vi "PLC WRITE DATA.vi"(8 "error in (no error)":errorcluster, 10 "cmd":string, 11 "TCP Network Connection in":refnum<k5>) -> (0 "error out":errorcluster, 3 "TCP Network Connection out":refnum<k5>)   [LabVIEW 2015]
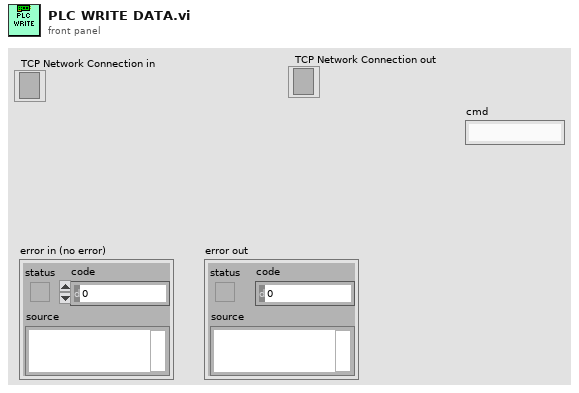
[diagram p1: front panel]
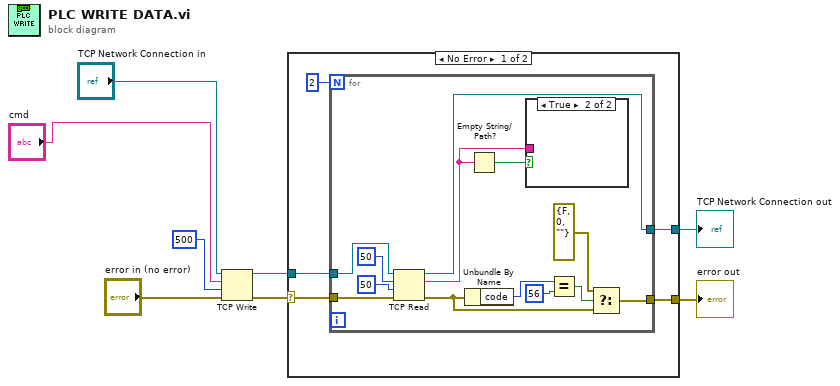
[diagram p0: block diagram]
diagram:
  n1 = TCP Write(connection ID="TCP Network Connection in", data in="cmd", error in (no error)="error in (no error)", 9:500 ("timeout ms (25000)")) -> (connection ID out=w2:refnum<k5>, error out=w3:errorcluster)  [unwired: 1 out]
  n2 = case shown="No Error" w3 {
    selector: w3 -> [w9 w27]
    tunnel: w2 -> [w13 w28]
    tunnel: [w11 w28] -> w4
    tunnel: [w10 w27] -> w7
    frame No Error {
      n3 = for {
        N: 2 ("Numeric 2") -> [_]
        tunnel: w13 -> [w26]
        tunnel: w9 -> [w25]
        tunnel: [w24] -> w11
        tunnel: [w15] -> w10
        n4 = TCP Read(connection ID=w26, bytes to read=50, error in (no error)=w25, 9:50 ("timeout ms (25000)")) -> (connection ID out=w24:refnum<k5>, data out=w20:string, error out=w16:errorcluster)  [unwired: 1 in]
        n5 = Unbundle By Name(w16) -> ("code"=w19:i32)
        n6 = Empty String/Path?(string/path=w20) -> (empty?=w21:bool)
        n7 = case shown="True" w21 {
          tunnel: w20 -> [_ _]
          frame False {
          }
          frame True {
          }
        }
        n8 = Equal?(x=w19, y=56) -> (x = y?=w17:bool)
        n9 = Select(t=errorcluster {"status"=FALSE, "code"=0, "source"=""}, s=w17, f=w16) -> (s? t:f=w15:errorcluster)
      }
    }
    frame Error {
    }
  }
  "error out" <- w7
  "TCP Network Connection out" <- w4
